vi "user_interface.vi"() -> ()   [LabVIEW 2019]
doc: "This example performs a serial port write and a serial port read. The parameters set for the serial port must match the parameters of the connected instrument or device. The VISA Configure Serial Port VI sets the configuration parameters. The front panel displays the controls used to configure the basic parameters, such as baud rate, data bits, and parity. The VI passes the VISA resource name to other VIs that perform operations on that VISA resource. The VISA Write function sends a command to the serial device and the VISA Read function returns data based on the command. The VISA Close function then closes the reference to the serial device. It is important to close the reference; otherwise, further communication through that port might not be possible."
uses:
  Arduino/Proteus/14_Arduino 328_LabView/Version_2015/Plantilla_Serial Folder/C/Program Files/National Instruments/LabVIEW 2016/examples/Instrument IO/Serial/support/Serial - Settings.ctl
  <vilib>/Instr/_visa.llb/VISA Configure Serial Port (Instr).vi
panel:
  out "Waveform Chart":i32(graph)
  out "Caudal":dbl(slide) caption="ml/min" scale=0.0..5000.0
  out "2B7":bool
  out "2B6":bool
  out "2B5":bool
  out "2B4":bool
  out "2B3":bool
  out "2B2":bool
  in  "stop":bool
  out "read buffer":string
  in  "byte count":u32=10
  in  "Serial Settings":T1={"baud rate"=9600, "data bits"=8, "parity"=enum."None", "stop bits"=10, "flow control"=0} {"flow control" items=["None"=0, "XON/XOFF"=1, "RTS/CTS"=2, "DTR/DSR"=4]; "stop bits" items=["1.0"=10, "1.5"=15, "2.0"=20]; "data bits" min=5 max=8 step=1; "baud rate" items=["75"=75, "110"=110, "134"=134, "150"=150, "300"=300, "600"=600, "1200"=1200, "1800"=1800, "2400"=2400, "4800"=4800, "7200"=7200, "9600"=9600, "14400"=14400, "19200"=19200, "28800"=28800, "38400"=38400, "56000"=56000, "57600"=57600, "115200"=115200, "128000"=128000, "230400"=230400]}
  in  "VISA resource name":refnum<visa-resource-name>="COM4"
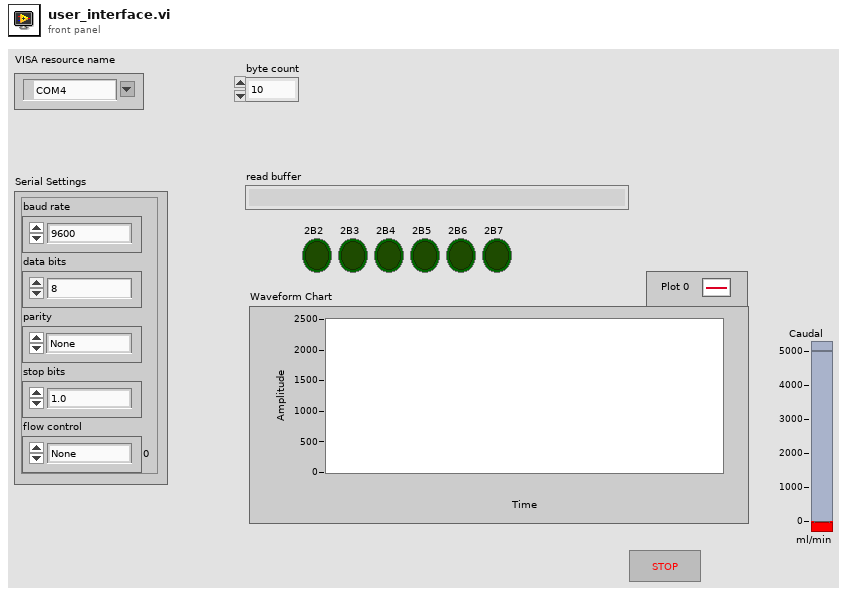
[diagram p1: front panel]
types:
  T1 = typedef "Serial - Settings.ctl" = cluster{"baud rate":u32, "data bits":u16, "parity":enum16{"None", "Odd", "Even", "Mark", "Space"}, "stop bits":u16, "flow control":u16}
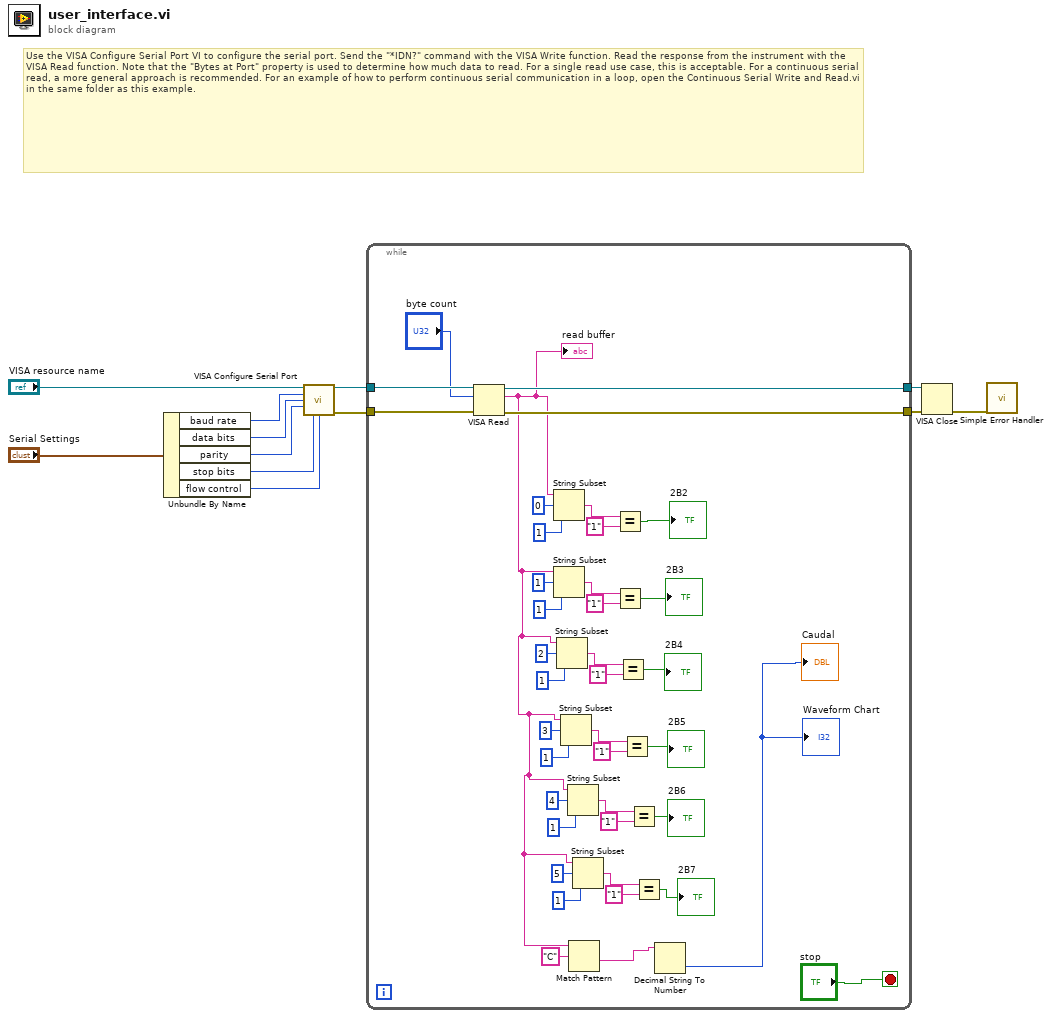
[diagram p0: block diagram]
diagram:
  # "Use the VISA Configure Serial Port VI to configure the serial port. Send the \"*IDN?\" command with the VISA Write function. Read the response from the instrument with the VISA Read function. Note that the \"Bytes at Port\" property is used to determine how much data to read. For a single read use case, this is acceptable. For a continuous serial read, a more general approach is recommended. For an example of how to perform continuous serial communication in a loop, open the Continuous Serial Write and Read.vi in the same folder as this example."
  n1 = Unbundle By Name "Unbundle By Name"("Serial Settings") -> ("baud rate"=w7:u32, "data bits"=w6:u16, "parity"=w5:enum16{"None", "Odd", "Even", "Mark", "Space"}, "stop bits"=w4:u16, "flow control"=w3:u16)
  n2 = call-poly "VISA Configure Serial Port"("VISA resource name"="VISA resource name", "baud rate (9600)"=w7, "data bits (8)"=w6, "parity (0:none)"=w5, "stop bits (10: 1 bit)"=w4, "flow control (0:none)"=w3) -> ("VISA resource name out"=w2:refnum<visa-resource-name>, "error out"=w1:errorcluster)  [unwired: 3 in, 5 out]
  n3 = while {
    tunnel: w2 -> [w50]
    tunnel: [w51] -> w10
    tunnel: w1 -> [w49]
    tunnel: [w52] -> w11
    stop <- "stop" stop-if-true
    n4 = VISA Read(VISA resource name=w50, byte count="byte count", error in (no error)=w49) -> (VISA resource name out=w51:refnum<visa-resource-name>, read buffer=w16:string, error out=w52:errorcluster)  [unwired: 1 out]
    "read buffer" <- w16
    n5 = String Subset(string=w16, offset (0)=0, length (rest)=1 ("length (rest)")) -> (substring=w44:string)
    n6 = String Subset(string=w16, offset (0)=1, length (rest)=1 ("length (rest)")) -> (substring=w40:string)
    n7 = String Subset(string=w16, offset (0)=2, length (rest)=1 ("length (rest)")) -> (substring=w34:string)
    n8 = String Subset(string=w16, offset (0)=3, length (rest)=1 ("length (rest)")) -> (substring=w31:string)
    n9 = String Subset(string=w16, offset (0)=4, length (rest)=1 ("length (rest)")) -> (substring=w26:string)
    n10 = Match Pattern(string=w16, regular expression="C") -> (after substring=w14:string)  [unwired: 1 in, 3 out]
    n11 = String Subset(string=w16, offset (0)=5, length (rest)=1 ("length (rest)")) -> (substring=w23:string)
    n12 = Equal?(x=w44, y="1") -> (x = y?=→"2B2":bool)
    n13 = Equal?(x=w40, y="1") -> (x = y?=→"2B3":bool)
    n14 = Equal?(x=w34, y="1") -> (x = y?=→"2B4":bool)
    n15 = Equal?(x=w31, y="1") -> (x = y?=→"2B5":bool)
    n16 = Equal?(x=w26, y="1") -> (x = y?=→"2B6":bool)
    n17 = Equal?(x=w23, y="1") -> (x = y?=→"2B7":bool)
    n18 = Decimal String To Number(string=w14) -> (number=→"Caudal" →"Waveform Chart":i32)  [unwired: 2 in, 1 out]
  }
  n19 = VISA Close(VISA resource name=w10, error in (no error)=w11) -> (error out=w9:errorcluster)
  n20 = call <vilib>:"Simple Error Handler.vi"("error in (no error)"=w9) -> ()  [unwired: 1 in, 8 out]
